vi "PIM Plot Measurement.vi"(0 "PIM Test Parameters":T3={"Stimulus"={"C1 Pwr dBm"=0.0, "C2 Pwr dBm"=0.0, "Power Units"=enum."dBm", "Meas Type"=enum."Time", "C1 Freq MHz"=0.0, "C2 Freq MHz"=0.0, "Swept Freq Step"=0}, "Measure"={"IM Order"=0, "Direction"=0, "Averaging"=1, "ALC ON?"=TRUE, "Peak Hold?"=TRUE, "Peak last N"=1, "Ref Level dBm"=-100.0, "Ref Units"=enum."dBm", "Num Samples"=1, "Sample units"=enum."Sample(s)", "Update Rate (s)"=0.0, "DUT PORT"=enum."Port 1", "Percent (%)"=100}, "Display"={"Power Scale"={"yRange_min"=0, "yRange_max"=0}, "xRange_span"=5}} {"Stimulus"."Swept Freq Step" items=[".2", ".4", "1.0", "2.0"]; "Measure"."Averaging" items=["None", "Minimum", "Normal", "High", "Maximum"]; "Measure"."Direction" items=["Reverse", "Forward", "Auxiliary"]; "Measure"."IM Order" items=["3rd", "5th", "7th", "9th", "11th", "13th", "15th", "17th", "19th", "21st", "23rd", "25th", "27th", "29th", "31st", "33rd"]}, 1 "Reset Plot?":bool, 2 "Freq Display Ref":refnum<vi>, 5 "TestSetDef":T1, 7 "Steps Per Sample":u32=1, 9 "Measurement Results":T2 {"IMPower_dBc(s)" format="%.2f"; "TxFreqs" format="%.2f"; "IMFreq(s)" format="%.2f"; "IMPower(s)" format="%.2f"; "TxPower" format="%.2f"}, 11 "error in (no error)":errorcluster, 12 "Sweep Sizes":i32[](array[numeric])) -> (3 "Point Plotted?":bool, 4 "Current Count":dbl, 6 "Percent Complete":dbl, 8 "Done?":bool, 10 "Discarded?":bool, 15 "error out":errorcluster)   [LabVIEW 2011]
uses:
  TypeDefs/PIM Test Parameters.ctl
  TypeDefs/PIM Stimulus Parameters.ctl
  SI.LIB/PIM.LIB/HW IO/PIM Sweep Step Size.ctl
  TypeDefs/PIM Measurement Parameters.ctl
  SI.LIB/PIM.LIB/HW IO/IMOrder.ctl
  SI.LIB/PIM.LIB/HW IO/MeasMode.ctl
  SI.LIB/PIM.LIB/HW IO/HW Averaging.ctl
  TypeDefs/PIM Meas Units.ctl
  SI.LIB/PIM.LIB/HW IO/DUTport.ctl
  TypeDefs/PIM Display Parameters.ctl
  drivers/PIM/PIM Results.ctl
  SI.LIB/PIM.LIB/HW IO/Test Set Definition.ctl
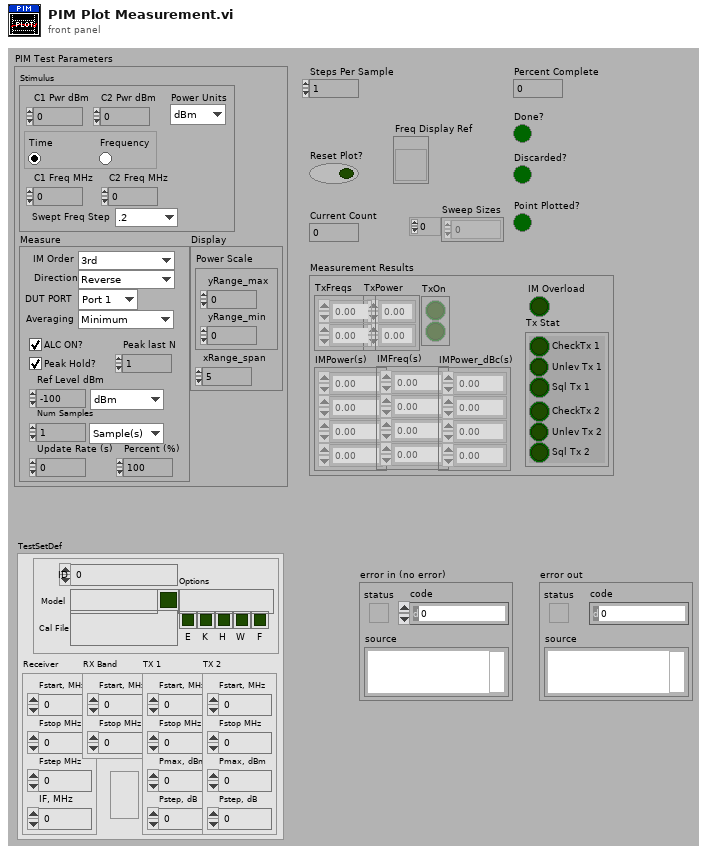
[diagram p1: front panel]
types:
  T1 = typedef "Test Set Definition.ctl" = cluster{"General":cluster{"ID":u32, "Model":string, "Dual Port?":bool, "Options":string, "Options":cluster{"E":bool, "K":bool, "H":bool, "W":bool, "F":bool}, "Cal File":path}, "Receiver":cluster{"Fstart, MHz":dbl, "Fstop MHz":dbl, "Fstep MHz":dbl, "IF, MHz":dbl}, "RX Band":cluster{"Fstart, MHz":dbl, "Fstop MHz":dbl}, "TX 1":cluster{"Fstart, MHz":dbl, "Fstop MHz":dbl, "Pmax, dBm":dbl, "Pstep, dB":dbl}, "TX 2":cluster{"Fstart, MHz":dbl, "Fstop MHz":dbl, "Pmax, dBm":dbl, "Pstep, dB":dbl}, "Low-side?":bool}
  T2 = typedef "PIM Results.ctl" = cluster{"TxFreqs":dbl[], "TxPower":dbl[], "TxOn":bool[], "IMPower(s)":dbl[], "IMFreq(s)":dbl[], "Tx Stat":cluster{"CheckTx 1":bool, "Unlev Tx 1":bool, "Sql Tx 1":bool, "CheckTx 2":bool, "Unlev Tx 2":bool, "Sql Tx 2":bool}, "IM Overload":bool, "IMPower_dBc(s)":dbl[]}
  T3 = typedef "PIM Test Parameters.ctl" = cluster{"Stimulus":T4, "Measure":T6, "Display":T12}
  T4 = typedef "PIM Stimulus Parameters.ctl" = cluster{"C1 Pwr dBm":dbl, "C2 Pwr dBm":dbl, "Power Units":enum16{"dBm", "Watts"}, "Meas Type":enum32{"Time", "Frequency"}, "C1 Freq MHz":dbl, "C2 Freq MHz":dbl, "Swept Freq Step":T5}
  T5 = typedef "PIM Sweep Step Size.ctl" = u16
  T6 = typedef "PIM Measurement Parameters.ctl" = cluster{"IM Order":T7, "Direction":T8, "Averaging":T9, "ALC ON?":bool, "Peak Hold?":bool, "Peak last N":u32, "Ref Level dBm":dbl, "Ref Units":enum16{"dBm", "dBc"}, "Num Samples":u32, "Sample units":T10, "Update Rate (s)":dbl, "DUT PORT":T11, "Percent (%)":u8}
  T7 = typedef "IMOrder.ctl" = u8
  T8 = typedef "MeasMode.ctl" = u16
  T9 = typedef "HW Averaging.ctl" = u16
  T10 = typedef "PIM Meas Units.ctl" = enum16{"Sample(s)", "Second(s)", "Sweep(s)"}
  T11 = typedef "DUTport.ctl" = enum16{"Port 1", "Port 2"}
  T12 = typedef "PIM Display Parameters.ctl" = cluster{"Power Scale":cluster{"yRange_min":i32, "yRange_max":i32}, "xRange_span":u32}
  T13 = cluster{"Start 1":dbl, "Stop 1":dbl, "Start 2":dbl, "Stop 2":dbl}
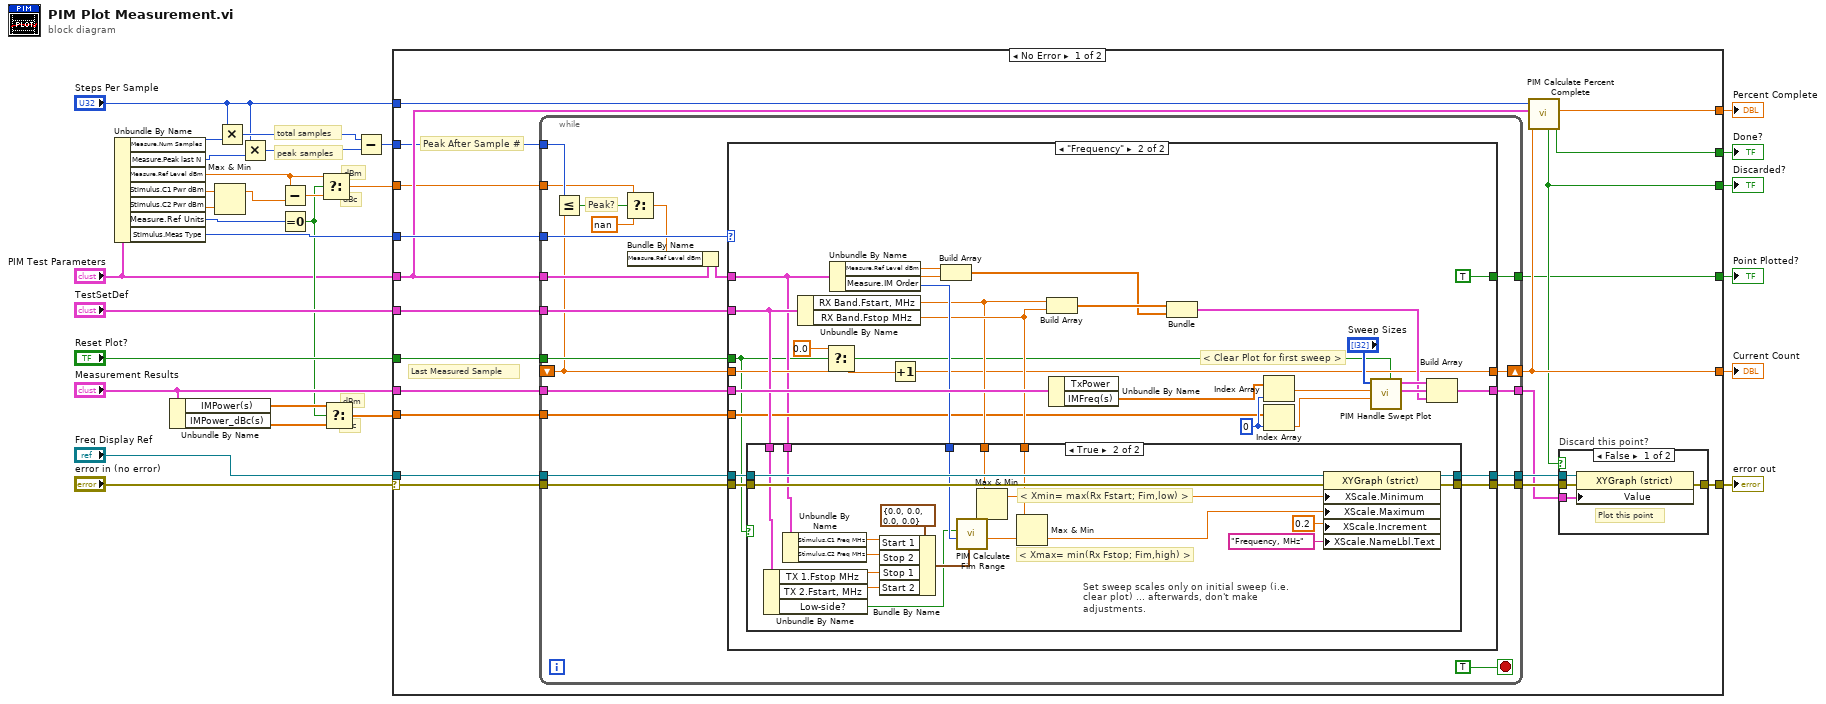
[diagram p0: block diagram]
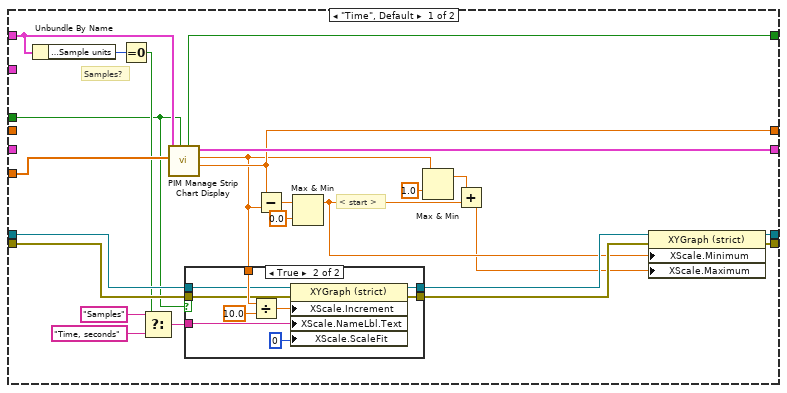
[diagram p3: hidden frame]
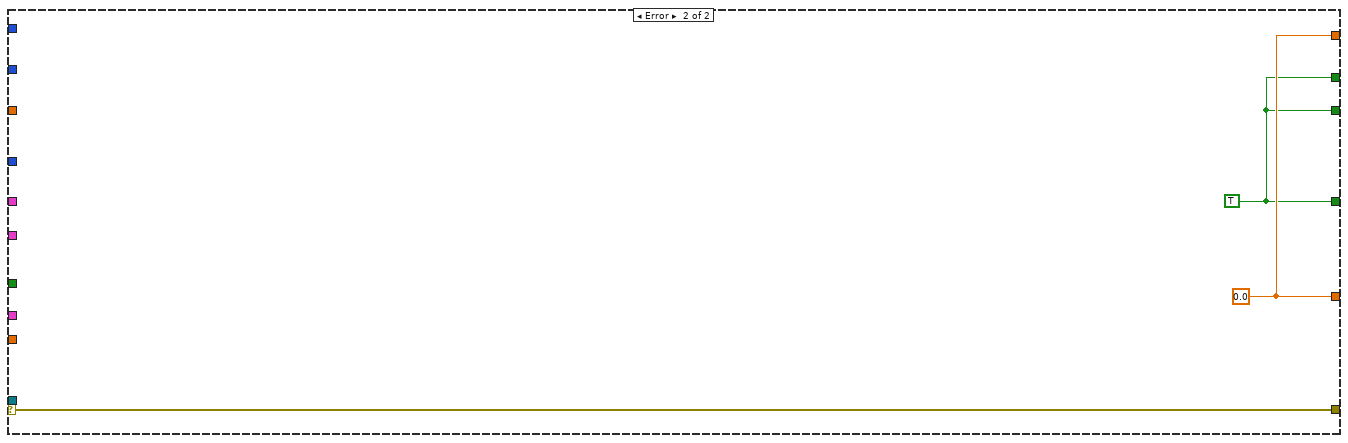
[diagram p6: hidden frame]
diagram:
  # "peak samples"
  # "total samples"
  # "dBc"
  # "dBm"
  # "dBc"
  # "dBm"
  n1 = Unbundle By Name("PIM Test Parameters") -> ("Measure.Num Samples"=w8:u32, "Measure.Peak last N"=w3:u32, "Measure.Ref Level dBm"=w21:dbl, "Stimulus.C1 Pwr dBm"=w23:dbl, "Stimulus.C2 Pwr dBm"=w22:dbl, "Measure.Ref Units"=w20:enum16{"dBm", "dBc"}, "Stimulus.Meas Type"=w19:enum32{"Time", "Frequency"})
  n2 = Unbundle By Name("Measurement Results") -> ("IMPower(s)"=w17:dbl[], "IMPower_dBc(s)"=w18:dbl[])
  n3 = Max & Min(x=w23, y=w22) -> (max(x,y)=w24:dbl)  [unwired: 1 out]
  n4 = Multiply(x="Steps Per Sample", y=w8) -> (x*y=w6:u32)
  n5 = Multiply(x="Steps Per Sample", y=w3) -> (x*y=w1:u32)
  n6 = Subtract(x=w21, y=w24) -> (x-y=w25:dbl)
  n7 = Equal To 0?(x=w20) -> (x = 0?=w15:bool)
  n8 = Select(t=w21, s=w15, f=w25) -> (s? t:f=w4:dbl)
  n9 = Select(t=w17, s=w15, f=w18) -> (s? t:f=w14:dbl[])
  n10 = Subtract(x=w6, y=w1) -> (x-y=w5:u32)
  n11 = case shown="No Error" "error in (no error)" {
    selector: "error in (no error)" -> [w40 w167]
    tunnel: "Reset Plot?" -> [w50 _]
    tunnel: "Freq Display Ref" -> [w47 _]
    tunnel: [w46 w167] -> w28
    tunnel: "TestSetDef" -> [w44 _]
    tunnel: [w39 w166] -> w26
    tunnel: w19 -> [w43 _]
    tunnel: "Measurement Results" -> [w42 _]
    tunnel: w14 -> [w41 _]
    tunnel: "PIM Test Parameters" -> [w38 _]
    tunnel: [w33 w165] -> w12
    tunnel: "Steps Per Sample" -> [w37 _]
    tunnel: [w36 w166] -> w11
    tunnel: [w35 w165] -> w10
    tunnel: [w34 w165] -> w9
    tunnel: w5 -> [w32 _]
    tunnel: w4 -> [w31 _]
    frame No Error {
      # "Last Measured Sample"
      # "Peak After Sample #"
      n12 = while {
        tunnel: w50 -> [w76]
        tunnel: [w75] -> w49
        tunnel: [w74] -> w48
        tunnel: w40 -> [w73]
        tunnel: w47 -> [w72]
        tunnel: [w71] -> w45
        tunnel: w44 -> [w70]
        tunnel: w38 -> [w63]
        tunnel: w43 -> [w69]
        tunnel: w42 -> [w68]
        shift-right: [w66] -> w39
        shift-left: _ -> [w60]
        tunnel: w41 -> [w65]
        tunnel: [w64] -> w33
        tunnel: w32 -> [w61]
        tunnel: w31 -> [w58]
        stop <- TRUE stop-if-true
        # "Peak?"
        n13 = Less Or Equal?(x=w61, y=w60) -> (x <= y?=w59:bool)
        n14 = Select(t=w58, s=w59, f=nan) -> (s? t:f=w56:dbl)
        n15 = Bundle By Name(cluster=w63, "Measure.Ref Level dBm"=w56) -> (w62:T3)
        n16 = case shown="\"Frequency\"" w69 {
          tunnel: w70 -> [_ w124]
          tunnel: w68 -> [_ w139]
          tunnel: w76 -> [w81 w112]
          tunnel: [w100 w132] -> w71
          tunnel: w72 -> [w96 w131]
          tunnel: w73 -> [w97 w130]
          tunnel: [w99 w129] -> w74
          tunnel: w62 -> [w89 w113]
          tunnel: [w98 w127] -> w75
          tunnel: [w90 w117] -> w66
          tunnel: w60 -> [_ w120]
          tunnel: w65 -> [w84 w115]
          tunnel: [w83 TRUE ("Point Plotted?")] -> w64
          frame "Time", Default {
            # "< start >"
            # "Samples?"
            n17 = Unbundle By Name(w89) -> ("Measure.Sample units"=w88:T10)
            n18 = Equal To 0?(x=w88) -> (x = 0?=w82:bool)
            n19 = Select(t="Samples" ("X Scale.Name Label.Text"), s=w82, f="Time, seconds" ("X Scale.Name Label.Text")) -> (s? t:f=w85:string)
            n20 = call "PIM Manage Strip Chart Display.vi"("Clear?"=w81, "IM Power(s)"=w84, "PIM Test Parameters"=w89) -> ("Strip Total Span (seconds|samples)"=w90:dbl, "Strip Window Span (seconds|samples)"=w78:dbl, "PIM Traces"=w100:cluster{"x-values":dbl[], "y-values":dbl[]}[], "Point Plotted?"=w83:bool)  [unwired: 5 out]
            n21 = case shown="True" w81 {
              tunnel: w78 -> [_ w110]
              tunnel: w97 -> [w101 w109]
              tunnel: [w101 w108] -> w93
              tunnel: [w102 w107] -> w92
              tunnel: w96 -> [w102 w106]
              tunnel: w85 -> [_ w103]
              frame False {
              }
              frame True {
                n22 = Divide(x=w110, y=10.0) -> (x/y=w105:dbl)
                n23 = property class="XYGraph (strict)"(reference=w106, error in=w109, "XScale.Increment"=w105, "XScale.NameLbl.Text"=w103, "XScale.ScaleFit"=u8 0 ("X Scale.Scale Fit")) -> (reference out=w107:refnum<vi>, error out=w108:errorcluster)
              }
            }
            n24 = Subtract(x=w90, y=w78) -> (x-y=w95:dbl)
            n25 = Max & Min(x=w95, y=0.0) -> (max(x,y)=w91:dbl)  [unwired: 1 out]
            n26 = Max & Min(x=w78, y=1.0) -> (max(x,y)=w79:dbl)  [unwired: 1 out]
            n27 = Add(x=w79, y=w91) -> (x+y=w77:dbl)
            n28 = property class="XYGraph (strict)"(reference=w92, error in=w93, "XScale.Minimum"=w91, "XScale.Maximum"=w77) -> (reference out=w98:refnum<vi>, error out=w99:errorcluster)
          }
          frame "Frequency" {
            w138 = 0 ("index")
            # "< Clear Plot for first sweep >"
            n29 = Unbundle By Name(w124) -> ("RX Band.Fstart, MHz"=w121:dbl, "RX Band.Fstop MHz"=w122:dbl)
            n30 = Select(t=0.0, s=w112, f=w120) -> (s? t:f=w118:dbl)
            n31 = Unbundle By Name(w113) -> ("Measure.Ref Level dBm"=w128:dbl, "Measure.IM Order"=w123:T7)
            n32 = case "Set sweep scales only on initial sweep (i.e. clear plot) ... afterwards, don't make adjustments." shown="True" w112 {
              tunnel: w131 -> [w141 w164]
              tunnel: w130 -> [w142 w163]
              tunnel: [w142 w162] -> w129
              tunnel: [w141 w161] -> w127
              tunnel: w124 -> [_ w160]
              tunnel: w123 -> [_ w155]
              tunnel: w122 -> [_ w154]
              tunnel: w121 -> [_ w151]
              tunnel: w113 -> [_ w148]
              frame False {
              }
              frame True {
                # "< Xmin= max(Rx Fstart; Fim,low) >"
                # "< Xmax= min(Rx Fstop; Fim,high) >"
                n33 = Unbundle By Name(w160) -> ("TX 1.Fstop MHz"=w158:dbl, "TX 2.Fstart, MHz"=w157:dbl, "Low-side?"=w143:bool)
                n34 = Unbundle By Name(w148) -> ("Stimulus.C1 Freq MHz"=w147:dbl, "Stimulus.C2 Freq MHz"=w146:dbl)
                n35 = Bundle By Name(cluster=T13 {"Start 1"=0.0, "Stop 1"=0.0, "Start 2"=0.0, "Stop 2"=0.0} ("Custom Sweep"), "Start 1"=w147, "Stop 2"=w146, "Stop 1"=w158, "Start 2"=w157) -> (w156:T13)
                n36 = call "PIM Calculate Fim Range.vi"("Custom Sweep"=w156, "Base Order (0)"=w155, "Low order IM? (T)"=w143) -> ("Fim, high"=w153:dbl, "Fim, low"=w150:dbl)  [unwired: 5 out]
                n37 = Max & Min(x=w151, y=w150) -> (max(x,y)=w149:dbl)  [unwired: 1 out]
                n38 = Max & Min(x=w154, y=w153) -> (min(x,y)=w152:dbl)  [unwired: 1 out]
                n39 = property class="XYGraph (strict)"(reference=w164, error in=w163, "XScale.Minimum"=w149, "XScale.Maximum"=w152, "XScale.Increment"=0.2 ("X Scale.Range:Increment"), "XScale.NameLbl.Text"="Frequency, MHz" ("X Scale.Name Label.Text")) -> (reference out=w161:refnum<vi>, error out=w162:errorcluster)
              }
            }
            n40 = Increment(x=w118) -> (x+1=w117:dbl)
            n41 = Build Array(w128, w128) -> (w116:dbl[])
            n42 = Build Array(w121, w122) -> (w140:dbl[])
            n43 = Unbundle By Name(w139) -> ("IMFreq(s)"=w126:dbl[])  [unwired: 1 out]
            n44 = Bundle(w140, w116) -> (w133:cluster{dbl[], dbl[]})  [unwired: 1 out]
            n45 = Index Array(array=w126, index=w138) -> (element=w137:dbl)
            n46 = Index Array(array=w115, index=w138) -> (element=w136:dbl)
            n47 = call "PIM Handle Swept Plot.vi"("Clear Plot? (f)"=w112, "IM Power"=w136, "IM Freq"=w137, "Sweep Sizes"="Sweep Sizes") -> ("F1 Up Trace"=w134:cluster{"new array":dbl[], "new array":dbl[]}, "F2 Down Trace"=w135:cluster{"new array":dbl[], "new array":dbl[]})  [unwired: 1 in, 3 out]
            n48 = Build Array(w135, w134, w133) -> (w132:cluster{"new array":dbl[], "new array":dbl[]}[])
          }
        }
      }
      n49 = call "PIM Calculate Percent Complete.vi"("Steps per sample"=w37, "Current Count"=w39, "PIM Test Parameters"=w38) -> ("Done?"=w35:bool, "% Complete"=w36:dbl, "Discard?"=w34:bool)  [unwired: 6 out]
      n50 = case "Discard this point?" shown="False" w34 {
        tunnel: w49 -> [w54 _]
        tunnel: w48 -> [w53 w55]
        tunnel: [w52 w55] -> w46
        tunnel: w45 -> [w51 _]
        frame False {
          # "Plot this point"
          n51 = property class="XYGraph (strict)"(reference=w54, error in=w53, "Value"=w51) -> (error out=w52:errorcluster)  [unwired: 1 out]
        }
        frame True {
        }
      }
    }
    frame Error {
      w166 = 0.0 ("Strip Total Span (seconds|samples)")
      w165 = TRUE ("Point Plotted?")
    }
  }
  "error out" <- w28
  "Current Count" <- w26
  "Point Plotted?" <- w12
  "Done?" <- w10
  "Percent Complete" <- w11
  "Discarded?" <- w9
